vi "Detector Set Config.vi"(8 "error in (no error)":errorcluster, 11 "PRIME Detector in":refnum<class "PRIME Detector.lvclass">) -> (0 "error out":errorcluster, 3 "PRIME Detector out":refnum<class "PRIME Detector.lvclass">)   [LabVIEW 2024, in "PRIME Detector.lvclass"]
uses:
  PRIME Detector.lvclass
  C:/Development/Prime-RIMAS/Detector/Detector Class/Detector Class.lvclass
  Detector Class.lvclass
  PRIME Detector.lvclass/PRIME Detector.ctl
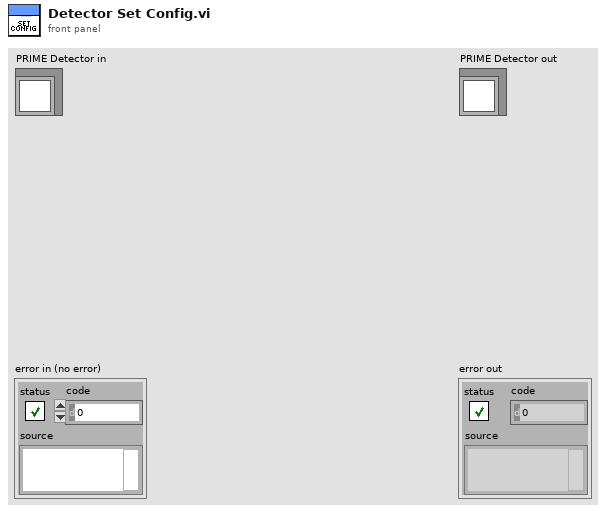
[diagram p1: front panel]
types:
  T1 = typedef "RIMAS Detector Config.ctl" = cluster{"Detector":u16, "Offsets":u16[][], "Detector Computer":T2, "FITS hdr template0":path, "FITS hdr template1":path, "FITS Data File Path":path, "FITS Detector Settings":T3, "Sim Folder":path, "Integration Mode":T4, "Integration Time":dbl, "Frame Int Time":dbl}
  T2 = typedef "RIMAS Detector Server Config.ctl" = cluster{"Machine":string, "Password":string, "FITS File Path":string, "Port":u16, "Header Path":string, "Name":string}
  T3 = typedef "RIMAS Observation Config.ctl" = cluster{"Exp Time Short":dbl, "# of Frames":dbl, "Exp Time Long":dbl, "# of Groups":dbl, "Object Name":string, "Object":string, "Obs Type":string, "Image Type":string, "Observer":string, "Observer Affiliation":string}
  T4 = typedef "Detector enum Detector Integration Mode.ctl" = enum16{"SSR", "CDS", "MEAN", "MEDIAN", "MODE", "MIIN", "MAX"}
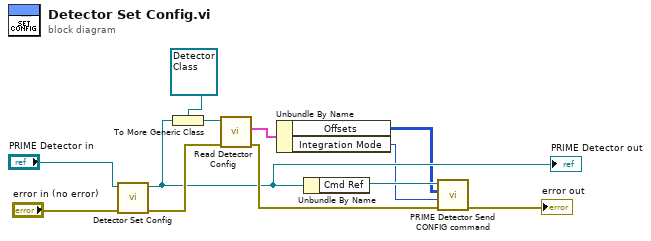
[diagram p0: block diagram]
diagram:
  n1 = call-parent "Detector Set Config.vi"("error in (no error)"="error in (no error)", "Detector Class in"="PRIME Detector in") -> ("error out"=w7:errorcluster, "Detector Class out"=w3:refnum<class "PRIME Detector.lvclass">)  [unwired: 8 in]
  "PRIME Detector out" <- w3
  n2 = To More Generic Class(target class=refnum<class "Detector Class.lvclass"> refnum ("Detector Class.lvclass"), reference=w3) -> (generic class reference=w9:refnum<class "Detector Class.lvclass">)
  n3 = call-dynamic "Read Detector Config.vi"("error in (no error)"=w7, "Detector Class in"=w9) -> ("error out"=w6:errorcluster, "Detector Config"=w8:T1)  [unwired: 7 in, 1 out]
  n4 = Unbundle By Name(w8) -> ("Offsets"=w2:u16[][], "Integration Mode"=w1:T4)
  n5 = Unbundle By Name(w3) -> ("Cmd Ref"=w5:refnum<k5>)
  n6 = call "PRIME Detector Send CONFIG command.vi"("error in (no error)"=w6, "Integration Mode"=w1, "Offsets"=w2, "connection ID"=w5) -> ("error out"=→"error out":errorcluster)  [unwired: 6 in, 1 out]
